vi "Python String to LabVIEW Data (I6 Array).vi"(8 "error in (no error)":errorcluster, 9 "type (I16 Array)":i16[](array[numeric]), 10 "Python String":string) -> (0 "error out":errorcluster, 2 "LabVIEW Data":i16[](array[numeric]))   [LabVIEW 2020, in "jki_python_data_tools.lvlib"]
doc: "Reads a value associated with key in a specified section of the configuration data identified by refnum. If \"key\" input is not specified, the name of the variant object is used as the key. the \"found?\" output will be TRUE for compount objects (clusters) only if all elements (recursively) are found.\n\nFor example a Boolean named \"Enable\" with a value of TRUE would correspond to the key-value pair:\n\nEnable=TRUE"
uses:
  jki_python_data_tools.lvlib
  Python String to LabVIEW Data (I16).vi
panel:
  # "Copyright © 2003-2009 JKI. All rights reserved.\n\nAuthor:\nPhilippe Guerit [philippe.guerit@jameskring.com]\nJim Kring [jim.kring@jameskring.com]\n\nThis library is provided \"AS IS\" ,WITHOUT WARRANTIES OR \nCONDITIONS OF ANY KIND, either express or implied.\n\nJames Kring, Inc. -- http://www.jameskring.com"
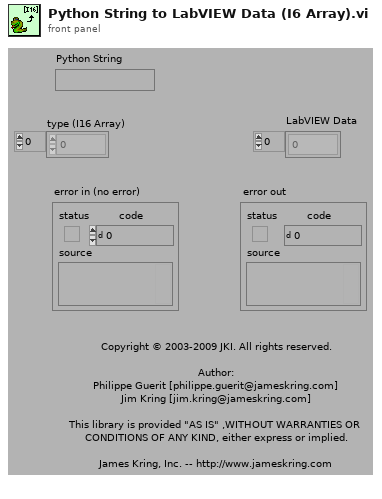
[diagram p1: front panel]
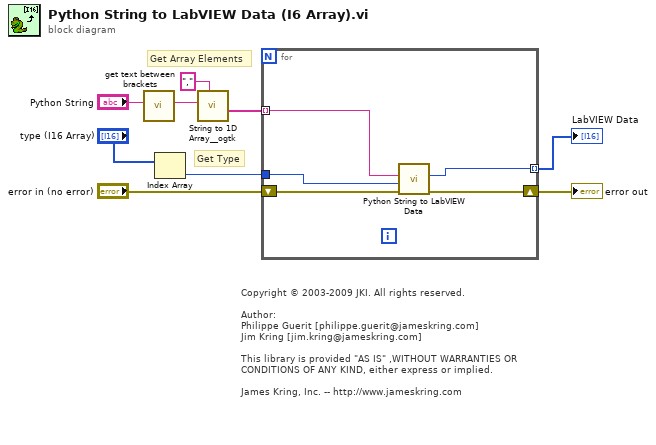
[diagram p0: block diagram]
diagram:
  # "Get Type"
  # "Get Array Elements"
  # "Copyright © 2003-2009 JKI. All rights reserved.\n\nAuthor:\nPhilippe Guerit [philippe.guerit@jameskring.com]\nJim Kring [jim.kring@jameskring.com]\n\nThis library is provided \"AS IS\" ,WITHOUT WARRANTIES OR \nCONDITIONS OF ANY KIND, either express or implied.\n\nJames Kring, Inc. -- http://www.jameskring.com"
  n1 = call "get text between brackets.vi"("Python String"="Python String") -> ("Text Between Brakets"=w3:string)  [unwired: 10 in]
  n2 = Index Array(array="type (I16 Array)") -> (element=w1:i16)  [unwired: 1 in]
  n3 = call <userlib>:"String to 1D Array__ogtk.vi"("delimiter (Tab)"=",", "string"=w3) -> ("Array of Strings"=w8:string[])  [unwired: 9 in]
  n4 = for {
    tunnel: [w11] -> w5 mode=indexing
    tunnel: w8 -> [w14] mode=indexing
    shift-right: [w12] -> w6
    shift-left: "error in (no error)" -> [w13]
    tunnel: w1 -> [w10]
    n5 = call-poly "Python String to LabVIEW Data.vi"("error in (no error)"=w13, "type (I16)"=w10, "Python String"=w14) -> ("error out"=w12:errorcluster, "LabVIEW Data"=w11:i16)  [unwired: 7 in]
  }
  "error out" <- w6
  "LabVIEW Data" <- w5
